vi "Microsync pin command.vi"(7 "Combo Box":string(combo)="PPL", 8 "error in (no error)":errorcluster, 10 "Arguments":T1, 11 "VISA resource name":refnum<visa-resource-name>) -> (0 "error out":errorcluster, 2 "return count":u32, 3 "VISA resource name out":refnum<visa-resource-name>)   [LabVIEW 2023]
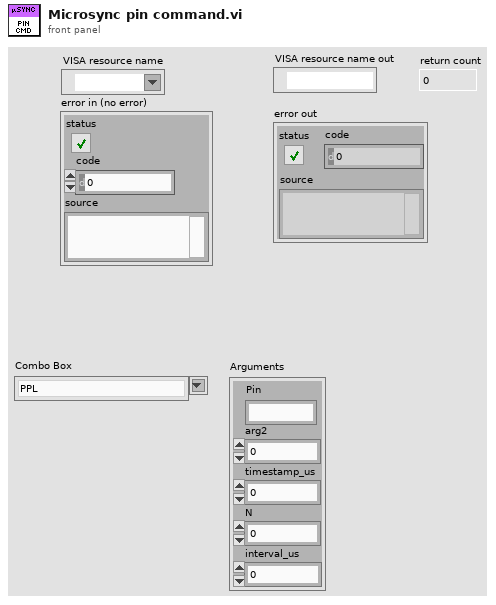
[diagram p1: front panel]
types:
  T1 = cluster{"interval_us":u32, "N":u32, "timestamp_us":u32, "arg2":u32, "Pin":string}
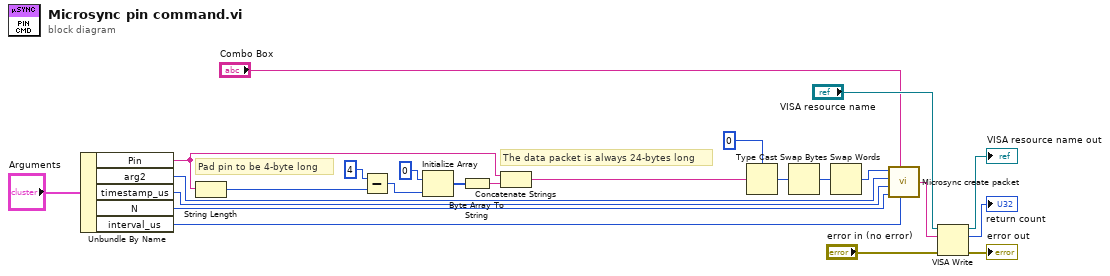
[diagram p0: block diagram]
diagram:
  # "Pad pin to be 4-byte long"
  # "The data packet is always 24-bytes long"
  n1 = Unbundle By Name("Arguments") -> ("Pin"=w4:string, "arg2"=w17:u32, "timestamp_us"=w16:u32, "N"=w15:u32, "interval_us"=w14:u32)
  n2 = String Length(string=w4) -> (length=w8:i32)
  n3 = Subtract(x=4, y=w8) -> (x-y=w7:i32)
  n4 = Initialize Array(u8 0 ("element"), w7) -> (w9:u8[])
  n5 = Byte Array To String(unsigned byte array=w9) -> (string=w10:string)
  n6 = Concatenate Strings(w4, w10) -> (w3:string)
  n7 = Type Cast(type=u32 0 ("arg1"), x=w3) -> (*(type *) &x=w12:u32)
  n8 = Swap Bytes(anything=w12) -> (byte swapped=w11:u32)
  n9 = Swap Words(1:w11) -> (0:w2:u32)
  n10 = call "Microsync create packet.vi"("interval_us"=w14, "Command"="Combo Box", "N"=w15, "timestamp_us"=w16, "arg2"=w17, "arg1"=w2) -> ("data packet"=w24:string)
  n11 = VISA Write(VISA resource name="VISA resource name", write buffer=w24, error in (no error)="error in (no error)") -> (VISA resource name out=→"VISA resource name out":refnum<visa-resource-name>, return count=→"return count":u32, error out=→"error out":errorcluster)
